vi "AnaBuse-Q2.vi"() -> ()   [LabVIEW 2019]
uses:
  <vilib>/Waveform/WDTOps.llb/WDT Get Waveform Subset DBL.vi
  <vilib>/measure/matone.llb/Extract Single Tone Information 1 Chan.vi
  <vilib>/measure/NI_MAPro.lvlib
panel:
  out "TEmpo de final \nda elevação 2":dbl format="%#_13g"
  out "TEmpo de inicio \nda elevação":dbl format="%#_13g"
  out "dt":dbl
  out "size(s)":i32
  out "detected amplitude":dbl format="%.2p"
  out "detected frequency":dbl format="%.2p"
  in  "Path":path
  out "ONDA TOTAL":waveform(dbl)[](graph)
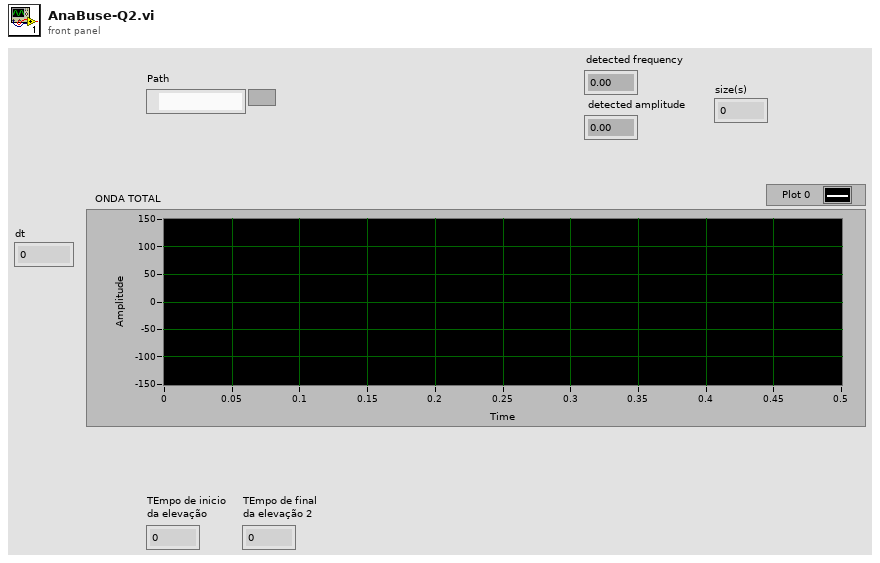
[diagram p1: front panel]
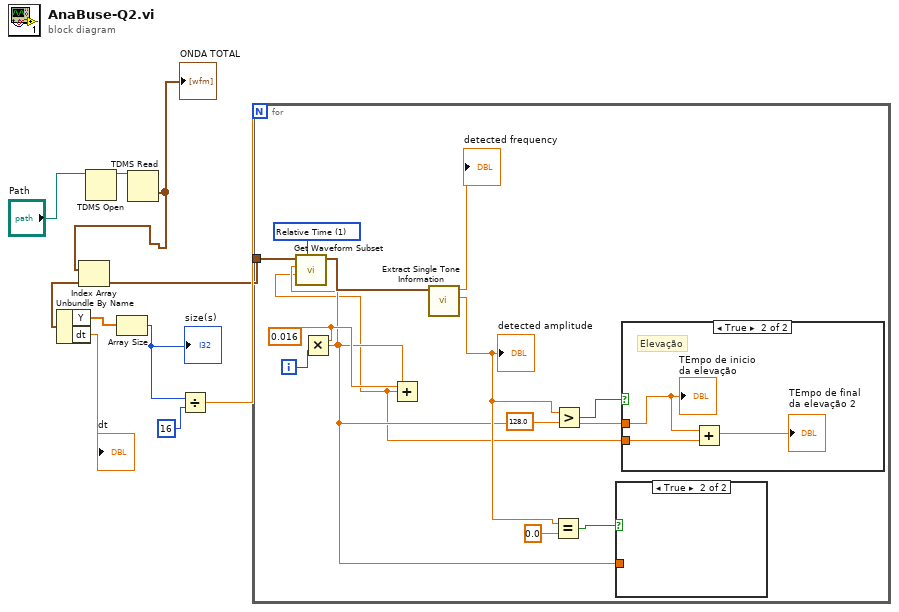
[diagram p0: block diagram]
diagram:
  n1 = TDMS Open(11:"Path") -> (3:w9:refnum<k34>)  [unwired: 6 in, 1 out]
  n2 = TDMS Read(0:w9) -> (10:w3:waveform(dbl)[])  [unwired: 7 in, 5 out]
  "ONDA TOTAL" <- w3
  n3 = Index Array(array=w3) -> (element=w2:waveform(dbl))  [unwired: 1 in]
  n4 = Unbundle By Name(w2) -> ("Y"=w4:dbl[], "dt"=→"dt":dbl)
  n5 = Array Size(array=w4) -> (size(s)=w7:i32)
  "size(s)" <- w7
  n6 = Divide(x=w7, y=16) -> (x/y=w5:dbl)
  n7 = for {
    N: w5 -> [_]
    tunnel: w2 -> [w17]
    i -> [w19]
    w18 = 0.016 ("duration")
    w22 = u16 1 items=["Samples", "Relative Time"] ("start/duration format")
    n8 = Multiply(x=w18, y=w19) -> (x*y=w11:dbl)
    n9 = Add(x=w18, y=w11) -> (x+y=w10:dbl)
    n10 = call-poly <vilib>:"Get Waveform Subset.vi"("start/duration format"=w22, "duration"=w10, "start samples/time"=w11, "waveform in"=w17) -> ("waveform out"=w21:waveform(dbl))  [unwired: 2 in, 3 out]
    n11 = call-poly <vilib>:"Extract Single Tone Information.vi"("time signal in"=w21) -> ("detected amplitude"=w13:dbl, "detected frequency"=→"detected frequency":dbl)  [unwired: 5 in, 4 out]
    "detected amplitude" <- w13
    n12 = Equal?(x=w13, y=0.0) -> (x = y?=w12:bool)
    n13 = Greater?(x=w13, y=128.0 ("detected amplitude")) -> (0:w16:bool)
    n14 = case shown="True" w12 {
      tunnel: w11 -> [_ _]
      frame False {
      }
      frame True {
      }
    }
    n15 = case shown="True" w16 {
      tunnel: w11 -> [_ w24]
      tunnel: w10 -> [_ w23]
      frame False {
      }
      frame True {
        # "Elevação"
        n16 = Add(x=w24, y=w23) -> (x+y=→"TEmpo de final \nda elevação 2":dbl)
        "TEmpo de inicio \nda elevação" <- w24
      }
    }
  }
